vi "Launch graph.vi"(8 "error in (no error)":errorcluster, 9 "Name":string, 10 "MagLabGraph.lvclass":refnum<class "MagLabGraph.lvclass">, 11 "Common Measurements in":refnum<class "Common Measurements.lvclass">) -> (0 "error out":errorcluster, 2 "Message Enqueuer out":refnum<class "Message Enqueuer.lvclass">, 3 "Common Measurements out":refnum<class "Common Measurements.lvclass">)   [LabVIEW 2015, in "Common Measurements.lvclass"]
uses:
  Common Measurements.lvclass
  Mag Lab Graph/MagLabGraph.lvclass
  <vilib>/ActorFramework/Message Enqueuer/Message Enqueuer.lvclass
  Common Measurements.lvclass/Common Measurements.ctl
  Mag Lab Graph/MagLabGraph.lvclass/MagLabGraph.ctl
  MagLabGraph Messages/Add file Msg/Add file Msg.lvclass/Add file Msg.ctl
  <vilib>/ActorFramework/Message Enqueuer/Message Enqueuer.lvclass/Message Enqueuer.ctl
  <vilib>/ActorFramework/Message Enqueuer/Enqueue.vi
  <vilib>/ActorFramework/Message Priority Queue/Priority Enqueue.vi
  Mag Lab Measure Controller/Mag Lab Measure Controller.lvclass
  MagLabGraph Messages/Add file Msg/Add file Msg.lvclass
  Mag Lab Error Handler/Mag Lab Error Handler.lvclass
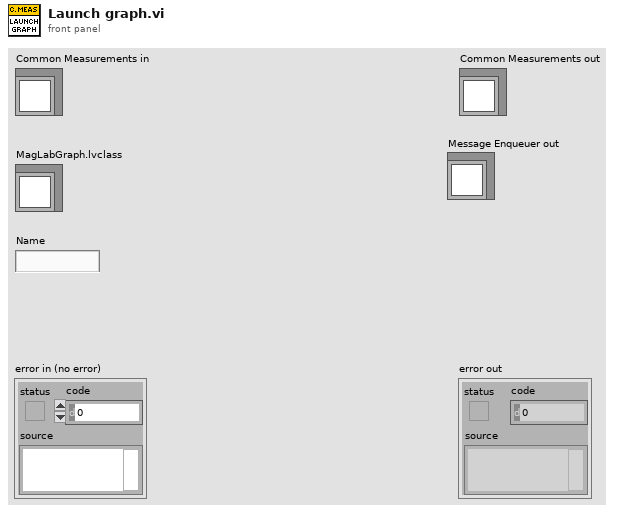
[diagram p1: front panel]
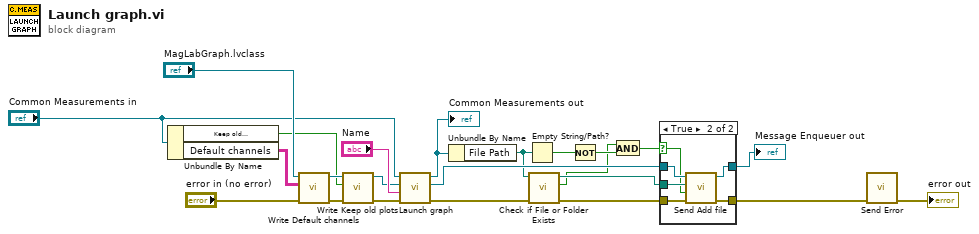
[diagram p0: block diagram]
diagram:
  n1 = Unbundle By Name("Common Measurements in") -> ("Keep old\nplots"=w3:bool, "Default channels"=w9:string[][])
  n2 = call "Write Default channels.vi"("error in (no error)"="error in (no error)", "Default channels"=w9, "MagLabGraph in"="MagLabGraph.lvclass") -> ("error out"=w5:errorcluster, "MagLabGraph out"=w7:refnum<class "MagLabGraph.lvclass">)  [unwired: 7 in]
  n3 = call "Write Keep old plots.vi"("error in (no error)"=w5, "Keep old plots"=w3, "MagLabGraph in"=w7) -> ("error out"=w4:errorcluster, "MagLabGraph out"=w6:refnum<class "MagLabGraph.lvclass">)  [unwired: 7 in]
  n4 = call-parent "Launch graph.vi"("error in (no error)"=w4, "Name"="Name", "MagLabGraph.lvclass"=w6, "Mag Lab Measure Base in"="Common Measurements in") -> ("error out"=w17:errorcluster, "Nested Actor's Enqueuer"=w21:refnum<class "Message Enqueuer.lvclass">, "Mag Lab Measure Base out"=w22:refnum<class "Common Measurements.lvclass">)  [unwired: 5 in]
  "Common Measurements out" <- w22
  n5 = Unbundle By Name(w22) -> ("File Path"=w16:path)
  n6 = Empty String/Path?(string/path=w16) -> (empty?=w15:bool)
  n7 = call <vilib>:"Check if File or Folder Exists.vi"("error in (no error)"=w17, "path"=w16) -> ("error out"=w18:errorcluster, "file or folder exists?"=w12:bool, "dup path"=w19:path)  [unwired: 7 in]
  n8 = Not(x=w15) -> (.not. x?=w13:bool)
  n9 = And(x=w12, y=w13) -> (x .and. y?=w14:bool)
  n10 = case shown="True" w14 {
    selector: w14 -> [_ w26]
    tunnel: w21 -> [w25 w31]
    tunnel: [w24 w30] -> w2
    tunnel: [w25 w29] -> w20
    tunnel: w19 -> [_ w28]
    tunnel: w18 -> [w24 w27]
    frame False {
    }
    frame True {
      n11 = call "Send Add file.vi"("error in (no error)"=w27, "Insert in front"=w26, "File Path Control"=w28, "Message Enqueuer"=w31) -> ("error out"=w30:errorcluster, "Message Enqueuer out"=w29:refnum<class "Message Enqueuer.lvclass">)  [unwired: 6 in]
    }
  }
  "Message Enqueuer out" <- w20
  n12 = call "Send Error.vi"("error in (no error)"=w2) -> ("error out"=→"error out":errorcluster)  [unwired: 9 in, 1 out]
